vi "classical_basis_matlab.vi"(0 "Encoding":cluster{"d":dbl, "y0":dbl, "y1":dbl}, 1 "c":dbl) -> (2 "modes":dbl[](array[numeric]), 3 "coeffs":dbl[](array[numeric]), 4 "phases":dbl[](array[numeric]))   [LabVIEW 2015]
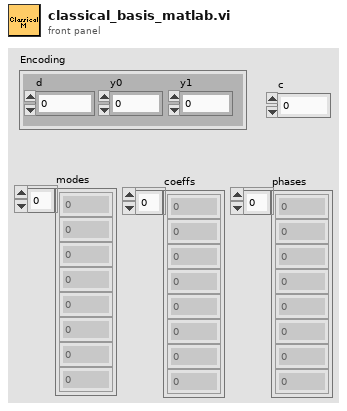
[diagram p1: front panel]
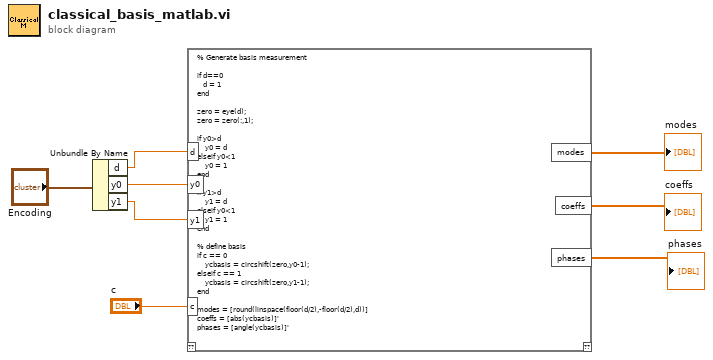
[diagram p0: block diagram]
diagram:
  n1 = Unbundle By Name("Encoding") -> ("d"=w3:dbl, "y0"=w2:dbl, "y1"=w1:dbl)
  n2 = script code="% Generate basis measurement\n\nif d==0\n   d = 1\nend\n\nzero = eye(d);\nzero = zero(:,1);\n\nif y0>d \n    y0 = d\nelseif y0<1\n    y0 = 1\nend\n\nif y1>d \n    y1 = d\nelseif y0<1\n    y1 = 1\nend\n\n% define basis\nif c == 0\n    ycbasis = circshift(zero,y0-1);\nelseif c == 1\n    ycbasis = circshift(zero,y1-1);\nend\n\nmodes = [round(linspace(floor(d/2),-floor(d/2),d))]\ncoeffs = [abs(ycbasis)]'\nphases = [angle(ycbasis)]'"("d"=w3, "c"="c", "y0"=w2, "y1"=w1) -> ("modes"=→"modes":dbl[], "coeffs"=→"coeffs":dbl[], "phases"=→"phases":dbl[])  [unwired: 1 in, 1 out]
